vi "Add Sink.vi"(6 "Include Encryption":bool=TRUE, 8 "Error In":errorcluster, 10 "Sinks":refnum<class "Log Sinks.lvclass">[](array[class]), 11 "Logger in":refnum<class "Log.lvclass">) -> (0 "Error Out":errorcluster, 3 "Logger":refnum<class "Log.lvclass">)   [LabVIEW 2019, in "TSC Event Logger.lvlib" / "Log.lvclass"]
doc: "Add a new sink to the list of Log Sinks\n\n-If include encryption is checked, it will apply the encryption from the first found non-default encryption method\n\n<b>Code Developed By:</b>\nTechnology Service Corporation\nBloomington, IN 47403\nwww.tsc.com/atcs\n\nDeveloper:\nDaniel Coons"
uses:
  Log.lvclass
  Log Sinks/Log Sinks.lvclass
  Log Sinks/Log Sinks.lvclass/Log Sinks.ctl
  Log.lvclass/Log.ctl
  Encryption/Encryption.lvclass
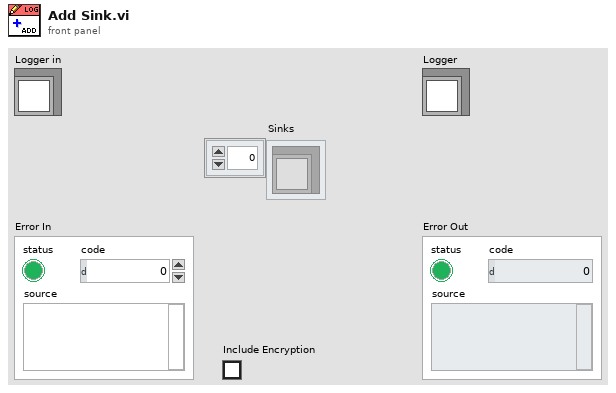
[diagram p1: front panel]
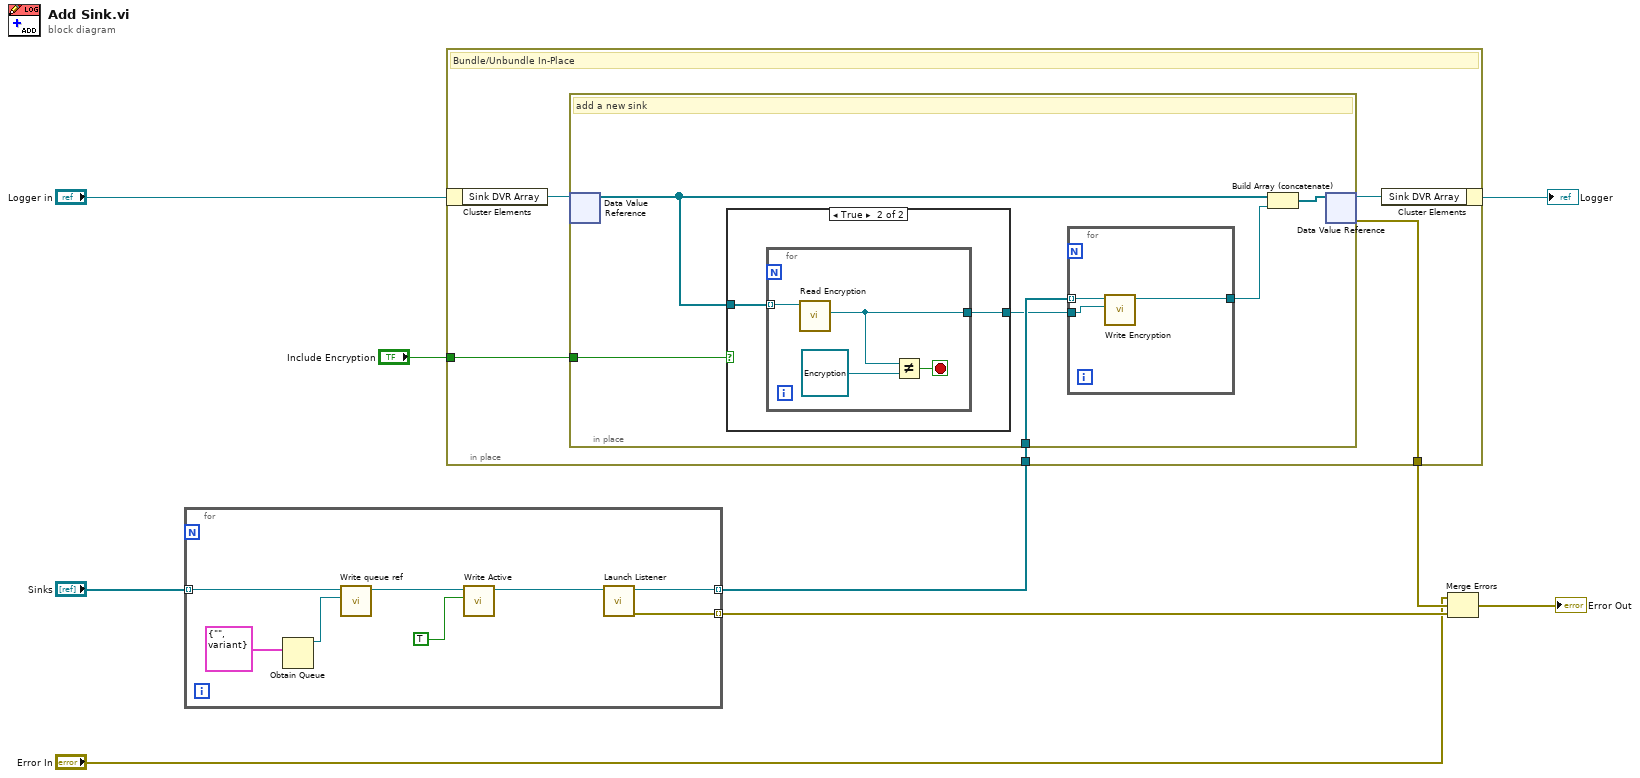
[diagram p0: block diagram]
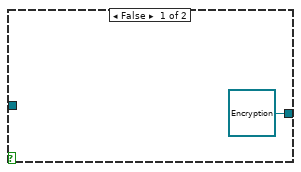
[diagram p2: hidden frame]
diagram:
  n1 = for {
    tunnel: [w16] -> w9 mode=indexing
    tunnel: [w10] -> w4 mode=indexing
    tunnel: "Sinks" -> [w15] mode=indexing
    n2 = Obtain Queue(element data type=cluster{"msg":string, "data":variant} {"msg"="", "data"=variant}) -> (queue out=w13:refnum<queue>)  [unwired: 4 in, 2 out]
    n3 = call "Write queue ref.vi"("queue ref"=w13, "Log Sinks in"=w15) -> ("Log Sinks out"=w14:refnum<class "Log Sinks.lvclass">)  [unwired: 9 in]
    n4 = call "Write Active.vi"("Active?"=TRUE, "Log Sinks in"=w14) -> ("Log Sinks out"=w12:refnum<class "Log Sinks.lvclass">)  [unwired: 9 in]
    n5 = call "Launch Listener.vi"("Log Sinks in"=w12) -> ("error out"=w16:errorcluster, "Log Sinks out"=w10:refnum<class "Log Sinks.lvclass">)  [unwired: 9 in]
  }
  n6 = in-place {
    in-place-border: w4 -> [w20]
    in-place-border: [w19] -> w3
    in-place-border: "Include Encryption" -> [w18]
    # "Bundle/Unbundle In-Place"
    n7 = in-place-cluster #1("Logger in") -> ("Sink DVR Array"=w22:refnum<data-value>)
    n8 = in-place {
      in-place-border: w20 -> [w28]
      in-place-border: w18 -> [w26]
      # "add a new sink"
      n9 = in-place-dvr #2(w22) -> (w25:refnum<class "Log Sinks.lvclass">[])  [unwired: 1 out]
      n10 = case shown="True" w26 {
        tunnel: w25 -> [_ w34]
        tunnel: [refnum<class "Encryption.lvclass"> refnum ("Encryption") w33] -> w23
        frame False {
        }
        frame True {
          n11 = for {
            tunnel: w34 -> [w38] mode=indexing
            tunnel: [w35] -> w33
            stop <- w36 stop-if-true
            n12 = call "Read Encryption.vi"("Log Sinks in"=w38) -> ("Encryption"=w35:refnum<class "Encryption.lvclass">)  [unwired: 8 in, 2 out]
            n13 = Not Equal?(x=w35, y=refnum<class "Encryption.lvclass"> refnum ("TSC Event Logger.lvlib:Encryption.lvclass")) -> (x != y?=w36:bool)
          }
        }
      }
      n14 = for {
        tunnel: w28 -> [w31] mode=indexing
        tunnel: [w30] -> w24
        tunnel: w23 -> [w29]
        n15 = call "Write Encryption.vi"("TSC Event Logger.lvlib:Encryption.lvclass"=w29, "Log Sinks in"=w31) -> ("Log Sinks out"=w30:refnum<class "Log Sinks.lvclass">)  [unwired: 8 in, 1 out]
      }
      n16 = Build Array (concatenate)(w25, w24) -> (w27:refnum<class "Log Sinks.lvclass">[])
      n17 = in-place-dvr #2(w27) -> (w21:refnum<data-value>, w19:errorcluster)
    }
    n18 = in-place-cluster #1("Sink DVR Array"=w21) -> (→"Logger":refnum<class "Log.lvclass">)
  }
  n19 = Merge Errors("Error In", w3, w9) -> (→"Error Out":errorcluster)
